vi "Write_signals_file.vi"(5 "Index":i32, 7 "Signal Array":T2[](array[typedef]), 8 "error in (no error)":errorcluster, 11 "ref":i32) -> (0 "error out":errorcluster, 3 "ref out":i32)   [LabVIEW 2013]
uses:
  Public API/Post_Signal.ctl
  Role ID.ctl
  Hardware ID.ctl
  Constraints.ctl
  <vilib>/addons/h5labview/polymorph/H5D_write_var.vi
  <vilib>/addons/h5labview/H5Dataset.lvlib
  <vilib>/addons/h5labview/H5GroupObject.lvlib
  <vilib>/addons/h5labview/H5Attrib.lvlib
panel:
  out "Role ID":T1
  # "Signal"
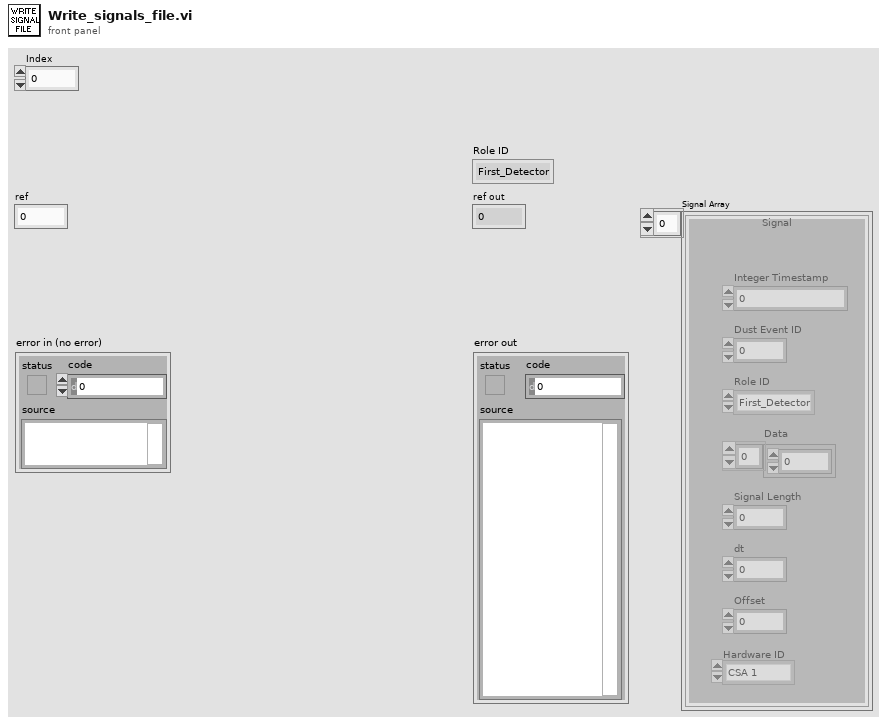
[diagram p1: front panel]
types:
  T1 = typedef "Role ID.ctl" = enum16{"First_Detector", "Second_Detector", "Third_Detector", "LeCroy_CH1", "LeCroy_CH2", "LeCroy_CH3", "LeCroy_CH4", "PSU"}
  T2 = typedef "Post_Signal.ctl" = cluster{"Integer Timestamp":i64, "Dust Event ID":i64, "Role ID":T1, "Data":sgl[], "Signal Length":i32, "dt":sgl, "Offset":dbl, "Hardware ID":T3}
  T3 = typedef "Hardware ID.ctl" = enum16{"Unknown", "CSA 1", "CSA 2", "CSA 3", "CSA 4", "CSA 5", "CSA 6"}
  T4 = typedef "Constraints.ctl" = cluster{"Upper Timestamp Range":timestamp, "Lower Timestamp Range":timestamp, "Experiment Group:":string, "Experiment Name:":i32[], "Upper Velocity Limit (km/s)":dbl, "Lower Velocity Limit (km/s)":dbl, "Upper Mass Limit (kg)":dbl, "Lower Mass Limit (kg)":dbl, "name array":string[], "Estimate Quality":cluster{dbl, dbl}}
  T5 = typedef "Query_Dust_Event.ctl" = cluster{"Dust Event ID":i64, "Integer Timestamp":i64, "Velocity":sgl, "Mass":sgl, "Charge":sgl, "Radius":sgl, "Passed_3rd_Detector":i8, "High Voltage":sgl, "+ High Voltage Supply":sgl, "- High Voltage Supply":sgl, "HV Control Difference":sgl, "Vacuum Pressure":sgl, "Radiation":sgl, "Column Current":sgl, "Lost Charge":sgl, "Chain Current":sgl, "Control High Voltage":sgl, "Current Group ID:":string, "Current Experiment Name:":string, "Current Experiment Description:":string, "Estimate Source":T6, "Estimate Quality":sgl, "File Location":T7, "Dust Type":string, "Dust Density":sgl}
  T6 = typedef "Estimate_source.ctl" = i8
  T7 = typedef "File_location.ctl" = i8
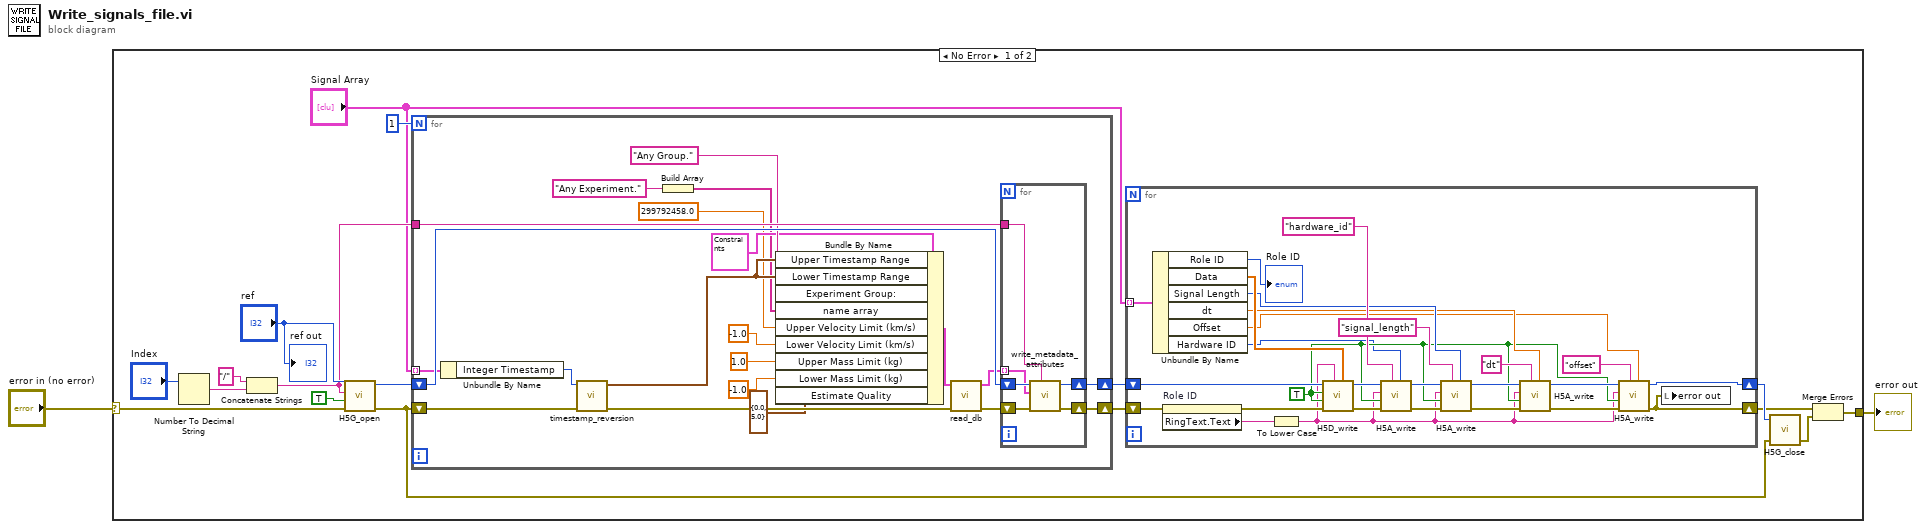
[diagram p0: block diagram]
diagram:
  n1 = case shown="No Error" "error in (no error)" {
    selector: "error in (no error)" -> [w17 w74]
    tunnel: [w4 w74] -> w1
    frame No Error {
      n2 = Number To Decimal String(number="Index") -> (decimal integer string=w15:string)  [unwired: 1 in]
      n3 = Concatenate Strings("/", w15) -> (w13:string)
      n4 = call <vilib>:"H5G_open.vi"("error in (no error)"=w17, "create? (F)"=TRUE, "name"=w13, "ref"="ref") -> ("error out"=w7:errorcluster, "group"=w12:i32)  [unwired: 2 in]
      n5 = for {
        N: 1 -> [_]
        tunnel: w13 -> [w31]
        shift-right: [w38] -> w10
        shift-left: w7 -> [w35]
        shift-right: [w39] -> w11
        shift-left: w12 -> [w40]
        tunnel: "Signal Array" -> [w29] mode=indexing
        n6 = Unbundle By Name(w29) -> ("Integer Timestamp"=w28:i64)
        n7 = call "timestamp_reversion.vi"("error in (no error)"=w35, "Integer Timestamp"=w28) -> ("error out"=w34:errorcluster, "time stamp"=w36:timestamp)  [unwired: 7 in]
        n8 = Build Array("Any Experiment.") -> (w21:string[])
        n9 = Bundle By Name(cluster=T4 {"Upper Timestamp Range"=timestamp(0 s since 1904-01-01), "Lower Timestamp Range"=timestamp(0 s since 1904-01-01), "Experiment Group:"="", "Experiment Name:"=[], "Upper Velocity Limit (km/s)"=0.0, "Lower Velocity Limit (km/s)"=0.0, "Upper Mass Limit (kg)"=0.0, "Lower Mass Limit (kg)"=0.0, "name array"=[], "Estimate Quality"={0.0, 0.0}} ("Constraints"), "Upper Timestamp Range"=w36, "Lower Timestamp Range"=w36, "Experiment Group:"="Any Group.", "name array"=w21, "Upper Velocity Limit (km/s)"=299792458.0 ("Upper Velocity Limit"), "Lower Velocity Limit (km/s)"=-1.0 ("Lower Velocity Limit"), "Upper Mass Limit (kg)"=1.0 ("Upper Mass Limit"), "Lower Mass Limit (kg)"=-1.0 ("Lower Mass Limit"), "Estimate Quality"=cluster{dbl, dbl} {0.0, 5.0} ("Dust Quality")) -> (w32:T4)
        n10 = call "read_db.vi"("error in (no error)"=w34, "Constraints"=w32) -> ("error out"=w33:errorcluster, "Dust Array"=w37:T5[])  [unwired: 5 in, 3 out]
        n11 = for {
          shift-right: [w45] -> w39
          shift-left: w40 -> [w46]
          shift-right: [w43] -> w38
          shift-left: w33 -> [w44]
          tunnel: w37 -> [w42] mode=indexing
          tunnel: w31 -> [w41]
          n12 = call "write_metadata_attributes.vi"("Group ID"=w41, "error in (no error)"=w44, "Cluster"=w42, "group ref"=w46) -> ("error out"=w43:errorcluster, "group ref out"=w45:i32)  [unwired: 4 in]
        }
      }
      n13 = for {
        tunnel: "Signal Array" -> [w70] mode=indexing
        shift-right: [w73] -> w18
        shift-left: w11 -> [w72]
        shift-right: [w71] -> w6
        shift-left: w10 -> [w51]
        w55 = TRUE ("preserve attribs?")
        n14 = Unbundle By Name(w70) -> ("Role ID"=→"Role ID":T1, "Data"=w69:sgl[], "Signal Length"=w63:i32, "dt"=w58:sgl, "Offset"=w53:dbl, "Hardware ID"=w52:T3)
        n15 = property on="Role ID" class="Enum (strict)"(error in=w51) -> (error out=w50:errorcluster, "RingText.Text"=w49:string)  [unwired: 1 in, 1 out]
        n16 = To Lower Case(string=w49) -> (all lower case string=w48:string)
        n17 = call-poly <vilib>:"H5D_write.vi"("data"=w69, "name"=w48, "error in (no error)"=w50, "overwrite?"=w55, "preserve attribs?"=w55, "ref"=w72) -> ("error out"=w67:errorcluster, "ref out"=w68:i32)  [unwired: 2 in]
        n18 = call <vilib>:"H5A_write.vi"("value"=w52, "attrib_name"="hardware_id", "error in (no error)"=w67, "overwrite? (F)"=w55, "obj_name"=w48, "ref"=w68) -> ("error out"=w65:errorcluster, "ref out"=w64:i32)  [unwired: 2 in]
        n19 = call <vilib>:"H5A_write.vi"("value"=w63, "attrib_name"="signal_length", "error in (no error)"=w65, "overwrite? (F)"=w55, "obj_name"=w48, "ref"=w64) -> ("error out"=w60:errorcluster, "ref out"=w61:i32)  [unwired: 2 in]
        n20 = call <vilib>:"H5A_write.vi"("value"=w58, "attrib_name"="dt", "error in (no error)"=w60, "overwrite? (F)"=w55, "obj_name"=w48, "ref"=w61) -> ("error out"=w56:errorcluster, "ref out"=w57:i32)  [unwired: 2 in]
        n21 = call <vilib>:"H5A_write.vi"("value"=w53, "attrib_name"="offset", "error in (no error)"=w56, "overwrite? (F)"=w55, "obj_name"=w48, "ref"=w57) -> ("error out"=w71:errorcluster, "ref out"=w73:i32)  [unwired: 2 in]
        n22 = local write "error out"(w71) -> ()
      }
      n23 = call <vilib>:"H5G_close.vi"("error in (no error)"=w7, "ref"=w18) -> ("error out"=w5:errorcluster)  [unwired: 3 in]
      n24 = Merge Errors(w6, w5) -> (w4:errorcluster)
      "ref out" <- "ref"
    }
    frame Error {
    }
  }
  "error out" <- w1
